vi "Probe (U256).vi"(9 "Data Valid":bool, 10 "Input":T1) -> (1 "Address":u64, 2 "Collected Data":T2(array[cluster]))   [LabVIEW 2011]
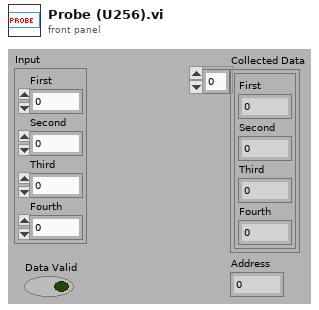
[diagram p1: front panel]
types:
  T1 = cluster{"First":u64, "Second":u64, "Third":u64, "Fourth":u64}
  T2 = cluster{"First":u64, "Second":u64, "Third":u64, "Fourth":u64}[]
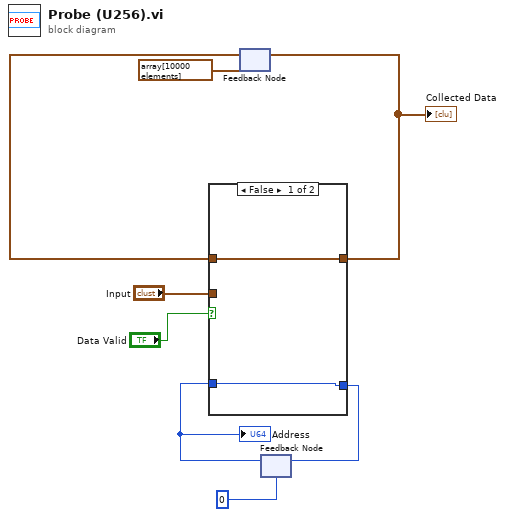
[diagram p0: block diagram]
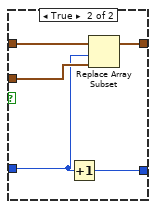
[diagram p2: hidden frame]
diagram:
  n1 = feedback #1(T2 array[10000 elements]) -> (w7:T2)
  n2 = feedback #2(u64 0) -> (w1:u64)
  "Address" <- w1
  n3 = case shown="False" "Data Valid" {
    tunnel: "Input" -> [_ w15]
    tunnel: w7 -> [w10 w14]
    tunnel: [w10 w13] -> w6
    tunnel: w1 -> [w9 w11]
    tunnel: [w9 w12] -> w3
    frame False {
    }
    frame True {
      n4 = Increment(x=w11) -> (x+1=w12:u64)
      n5 = Replace Array Subset(array=w14, new element=w15, index=w11) -> (w13:T2)
    }
  }
  "Collected Data" <- w6
  n6 = feedback-in #1(w6) -> ()
  n7 = feedback-in #2(w3) -> ()
